vi "Texture Defect Detection.vi"() -> ()   [LabVIEW 2014]
doc: "This example shows how to use the texture defect detection VI in NI Vision.\n\nTexture defect detection identifies areas of the image presentating a significantly different texture. First, use the Texture Training Interface to teach your application a reference texture. The Texture Training Interface creates a texture classifier file, which you then use to detect texture defects."
uses:
  <vilib>/vision/NI_Vision_Development_Module.lvlib
panel:
  out "Number of Defects":i32
  in  "Stop":bool
  in  "Delay (s.)":dbl(slide)=1.008 scale=0.0..2.0
  out "Image":T1(plugin-control)
  # "Overview: Demonstrates detecting texture defects.\nRequirements: NI Vision Development Module\nInstructions: Run the VI."
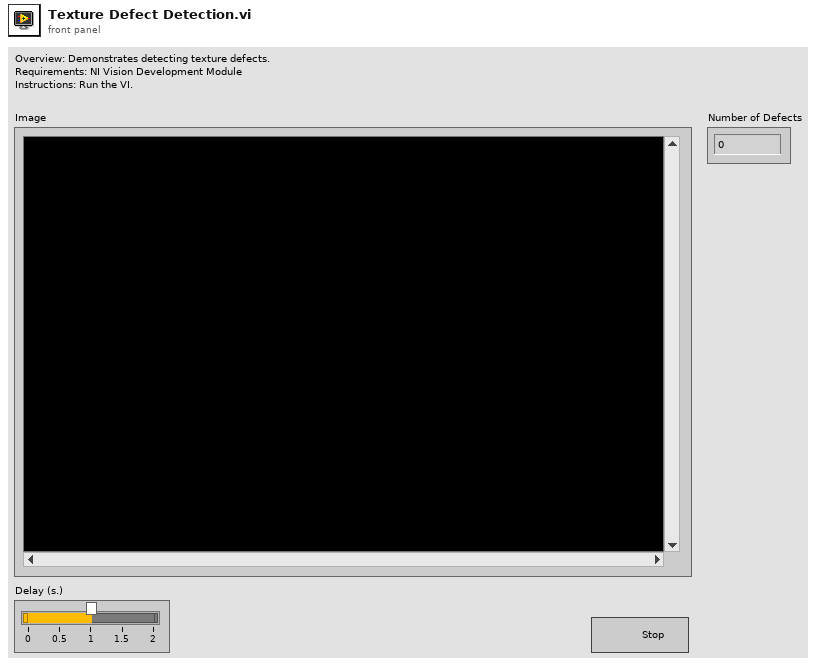
[diagram p1: front panel]
types:
  T1 = typedef "IMAQ Image.ctl" = refnum<image>
  T2 = typedef "IMAQ Classifier Session.ctl" = refnum<k1>
  T3 = typedef "ROI Descriptor" = cluster{"Global Rectangle":i32[], "Contours":cluster{"ID":enum32{"External", "Internal"}, "Type":u32, "Coordinates":i32[]}[]}
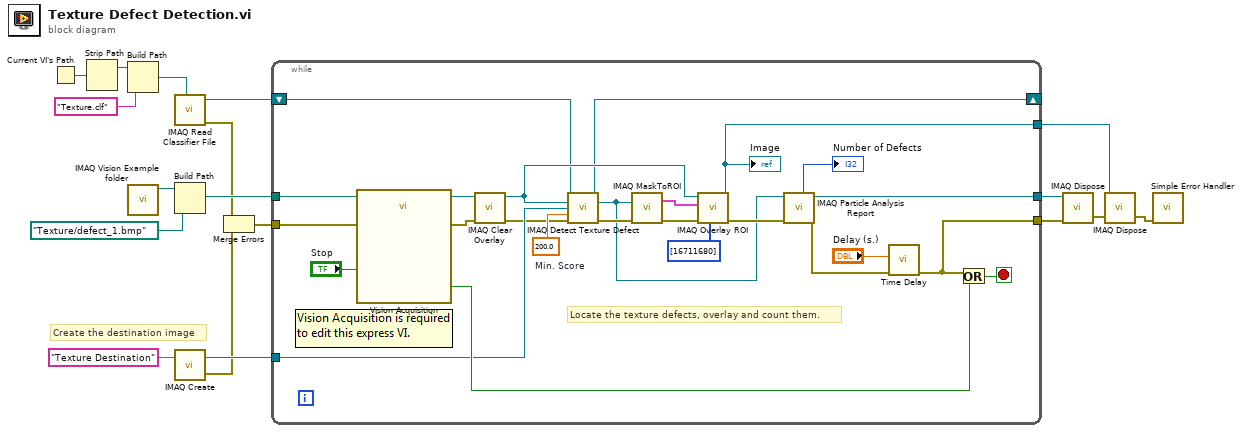
[diagram p0: block diagram]
diagram:
  # "Create the destination image"
  n1 = Current VI's Path() -> (path=w12:path)
  n2 = Strip Path(path=w12) -> (stripped path=w13:path)  [unwired: 1 out]
  n3 = Build Path(base path=w13, name or relative path="Texture.clf") -> (appended path=w11:path)
  n4 = call "IMAQ Vision Example folder.vi"() -> ("Example Image Path"=w18:path)  [unwired: 11 in]
  n5 = call "IMAQ Read Classifier File"("File Path"=w11) -> ("error out"=w3:errorcluster, "Classifier Session"=w7:T2)  [unwired: 3 in, 6 out]
  n6 = Build Path(base path=w18, name or relative path=path "Texture/defect_1.bmp") -> (appended path=w16:path)
  n7 = call "IMAQ Create"("Image Name"="Texture Destination") -> ("New Image"=w8:T1, "error out"=w2:errorcluster)  [unwired: 3 in, 1 out]
  n8 = Merge Errors(w3, w2) -> (w1:errorcluster)
  n9 = while {
    tunnel: w16 -> [w41]
    tunnel: [w27] -> w15
    tunnel: [w37] -> w14
    tunnel: w8 -> [w23]
    shift-right: [w25] -> _
    shift-left: w7 -> [w26]
    tunnel: [w20] -> w4
    tunnel: w1 -> [w19]
    stop <- w38 stop-if-true
    w36 = 200.0  # Min. Score
    # "Locate the texture defects, overlay and count them."
    n10 = call "Vision Acquisition"("Image Path"=w41, "Stop (F)"="Stop", "error in"=w19) -> ("Image Out"=w24:T1, "Stopped"=w39:bool, "error out"=w40:errorcluster)  [unwired: 22 in]
    n11 = call "IMAQ Clear Overlay"("error in (no error)"=w40, "Image"=w24) -> ("error out"=w21:errorcluster, "Image Out"=w30:T1)  [unwired: 1 in, 7 out]
    n12 = call "IMAQ Detect Texture Defect"("Classifier Session"=w26, "Image Src"=w30, "Image Dst"=w23, "Min. Defect Identification Score"=w36, "error in (no error)"=w21) -> ("Classifier Session (dup)"=w25:T2, "Image Dst Out"=w22:T1, "error out"=w31:errorcluster)  [unwired: 4 in, 4 out]
    n13 = call "IMAQ MaskToROI"("Image"=w22, "error in (no error)"=w31) -> ("ROI Descriptor"=w33:T3, "error out"=w32:errorcluster)  [unwired: 2 in, 4 out]
    n14 = call "IMAQ Overlay ROI"("Colors (Green)"=u32[] [16711680], "error in (no error)"=w32, "ROI Descriptor"=w33, "Image"=w30) -> ("error out"=w35:errorcluster, "Image Out"=w20:T1)  [unwired: 2 in, 4 out]
    "Image" <- w20
    n15 = call "IMAQ Particle Analysis Report"("error in (no error)"=w35, "Image"=w22) -> ("error out"=w29:errorcluster, "Image Out (duplicate)"=w27:T1, "Number of Particles"=→"Number of Defects":i32)  [unwired: 1 in, 6 out]
    n16 = call "Time Delay"("error in (no error)"=w29, "Delay Time (s)"="Delay (s.)") -> ("error out"=w37:errorcluster)  [unwired: 9 in]
    n17 = Or(x=w37, y=w39) -> (x .or. y?=w38:bool)
  }
  n18 = call "IMAQ Dispose"("Image"=w15, "error in (no error)"=w14) -> ("error out"=w6:errorcluster)  [unwired: 1 in, 3 out]
  n19 = call "IMAQ Dispose"("Image"=w4, "error in (no error)"=w6) -> ("error out"=w5:errorcluster)  [unwired: 1 in, 3 out]
  n20 = call <vilib>:"Simple Error Handler.vi"("error in (no error)"=w5) -> ()  [unwired: 4 in, 5 out]
